vi "test-vi-1-validate.vi"(8 "error in (no error)":errorcluster, 11 "VI in":refnum<vi>) -> (0 "error out":errorcluster, 2 "ClassName":string, 3 "VI out":refnum<vi>)   [LabVIEW 2016, in "test-find-vi-by-name.lvlib"]
uses:
  test-find-vi-by-name.lvlib
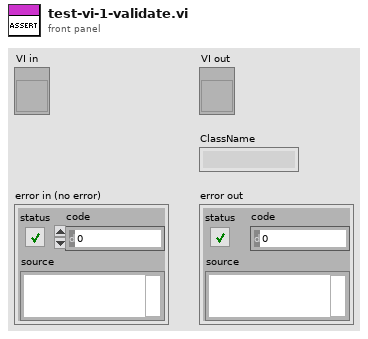
[diagram p1: front panel]
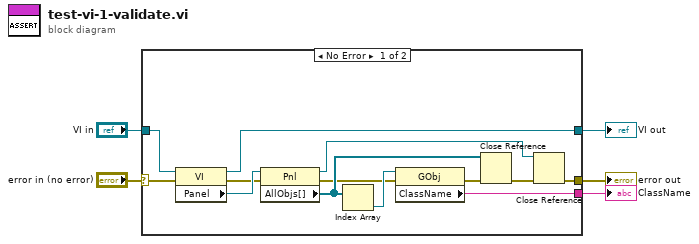
[diagram p0: block diagram]
diagram:
  n1 = case shown="No Error" "error in (no error)" {
    selector: "error in (no error)" -> [w6 w20]
    tunnel: [w16 _] -> w5
    tunnel: [w13 w19] -> w4
    tunnel: [w11 w20] -> w3
    tunnel: "VI in" -> [w8 w19]
    frame No Error {
      n2 = property class="VI"(reference=w8, error in=w6) -> (reference out=w13:refnum<vi>, error out=w7:errorcluster, "Panel"=w10:refnum<vi>)
      n3 = property class="Pnl"(reference=w10, error in=w7) -> (reference out=w12:refnum<vi>, error out=w9:errorcluster, "AllObjs[]"=w18:refnum<vi>[])
      n4 = Index Array(array=w18) -> (element=w15:refnum<vi>)  [unwired: 1 in]
      n5 = property class="GObj"(reference=w15, error in=w9) -> (error out=w14:errorcluster, "ClassName"=w16:string)  [unwired: 1 out]
      n6 = Close Reference(reference=w18, error in (no error)=w14) -> (error out=w17:errorcluster)
      n7 = Close Reference(reference=w12, error in (no error)=w17) -> (error out=w11:errorcluster)
    }
    frame Error {
    }
  }
  "ClassName" <- w5
  "VI out" <- w4
  "error out" <- w3
